vi "2015 INI Loader.vi"() -> (1 "Inches Per Tick":dbl=0.103 format="%.4f", 2 "Gyro 1 Center Voltage":dbl format="%.4f", 3 "Gyro 1 Gain":dbl format="%.4f", 5 "Turn PID gains":T1={"proportional gain (Kc)"=0.015999999999999997, "integral time (Ti, min)"=0.01800000000000001, "derivative time (Td, min)"=0.0} {"proportional gain (Kc)" min=0.0 max=1.0 step=0.001; "integral time (Ti, min)" min=0.0 max=1.0 step=0.001}, 6 "Elevator PID gains":T1={"proportional gain (Kc)"=1.0, "integral time (Ti, min)"=0.01, "derivative time (Td, min)"=0.0} {"derivative time (Td, min)" format="%.3f"; "integral time (Ti, min)" format="%.3f"; "proportional gain (Kc)" format="%.3f"}, 7 "Base PID gains":T1 {"derivative time (Td, min)" format="%.3f"; "integral time (Ti, min)" format="%.3f"; "proportional gain (Kc)" format="%.3f"})   [LabVIEW 2014]
uses:
  PID Typdef.ctl
  <vilib>/Utility/config.llb/Read Key (Double).vi
  <vilib>/Rock Robotics/Network Tables/SD Write String.vi
  <vilib>/Utility/config.llb/NI_LVConfig.lvlib
panel:
  out "ED":dbl
  out "EI":dbl
  out "EP":dbl
  out "TD":dbl
  out "TI":dbl
  out "TP":dbl
  out "BED":dbl
  out "BEI":dbl
  out "BEP":dbl
  out "path":path
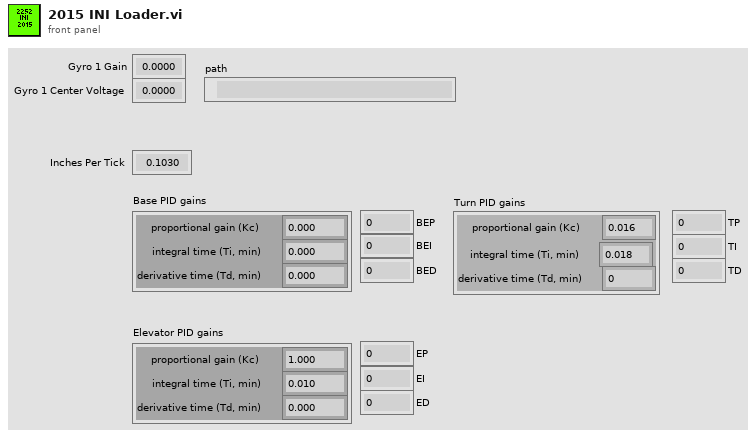
[diagram p1: front panel]
types:
  T1 = cluster{"proportional gain (Kc)":dbl, "integral time (Ti, min)":dbl, "derivative time (Td, min)":dbl}
  T2 = typedef "PID Typdef.ctl" = cluster{"proportional gain (Kc)":dbl, "integral time (Ti, min)":dbl, "derivative time (Td, min)":dbl}
  T3 = typedef "NI_LVConfig.lvlib/Config Data RefNum.ctl" = refnum<k1>
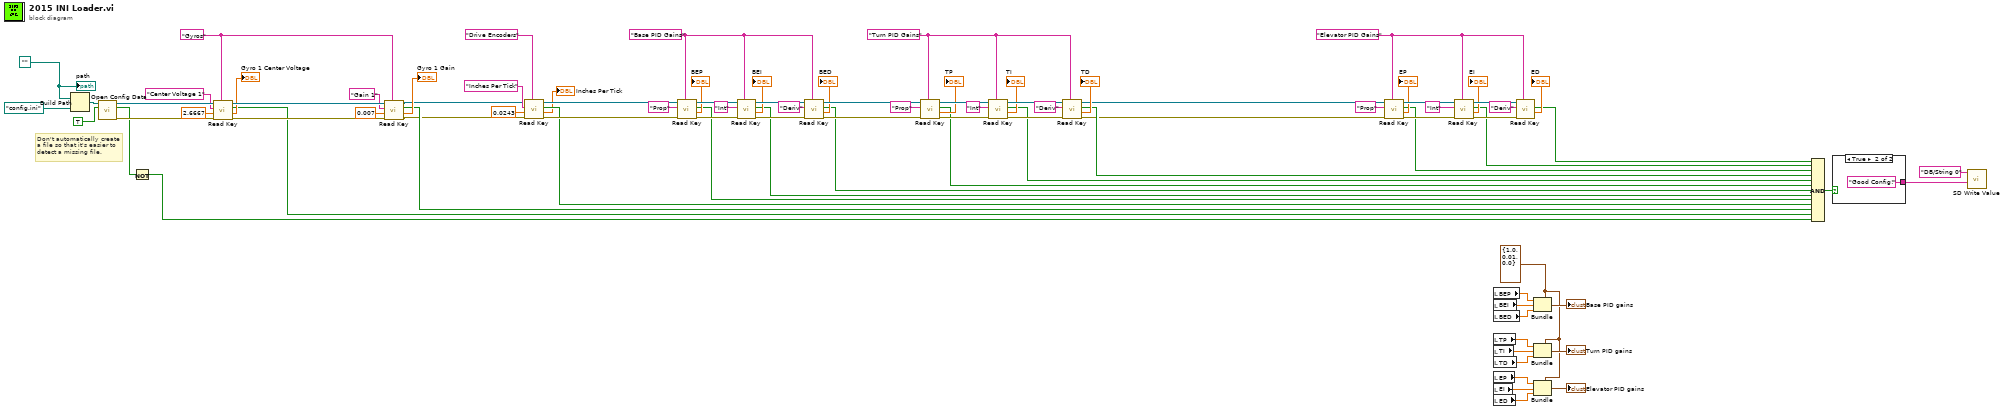
[diagram p0: block diagram]
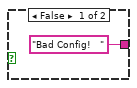
[diagram p2: hidden frame]
diagram:
  w3 = path ""
  w62 = T2 {"proportional gain (Kc)"=1.0, "integral time (Ti, min)"=0.01, "derivative time (Td, min)"=0.0} ("PID Typedef")
  w41 = "Elevator PID Gains" ("section")
  w44 = "Turn PID Gains" ("section")
  w53 = "Base PID Gains" ("section")
  w77 = "Gyros" ("section")
  # "Don't automatically create\na file so that it's easier to\ndetect a missing file."
  n1 = Build Path(base path=w3, name or relative path=path "config.ini" ("configuration file path")) -> (appended path=w89:path)
  n2 = call <vilib>:"Open Config Data.vi"("create file if necessary (T)"=TRUE, "configuration file path"=w89) -> ("error out"=w88:errorcluster, "file created?"=w81:bool, "refnum"=w87:T3)  [unwired: 7 in]
  n3 = Not(x=w81) -> (.not. x?=w69:bool)
  n4 = call-poly <vilib>:"Read Key.vi"("section"=w77, "error in (no error)"=w88, "default value"=2.6667, "key"="Center Voltage 1", "refnum"=w87) -> ("error out"=w84:errorcluster, "value"=→"Gyro 1 Center Voltage":dbl, "found?"=w70:bool, "refnum out"=w83:T3)  [unwired: 3 in]
  n5 = call-poly <vilib>:"Read Key.vi"("section"=w77, "error in (no error)"=w84, "default value"=0.007, "key"="Gain 1", "refnum"=w83) -> ("error out"=w66:errorcluster, "value"=→"Gyro 1 Gain":dbl, "found?"=w71:bool, "refnum out"=w65:T3)  [unwired: 3 in]
  n6 = call-poly <vilib>:"Read Key.vi"("section"="Drive Encoders", "error in (no error)"=w66, "default value"=0.0243, "key"="Inches Per Tick", "refnum"=w65) -> ("error out"=w60:errorcluster, "value"=→"Inches Per Tick":dbl, "found?"=w14:bool, "refnum out"=w59:T3)  [unwired: 3 in]
  n7 = call-poly <vilib>:"Read Key.vi"("section"=w53, "error in (no error)"=w60, "key"="Prop", "refnum"=w59) -> ("error out"=w49:errorcluster, "value"=→"BEP":dbl, "found?"=w13:bool, "refnum out"=w58:T3)  [unwired: 4 in]
  n8 = call-poly <vilib>:"Read Key.vi"("section"=w53, "error in (no error)"=w49, "key"="Int", "refnum"=w58) -> ("error out"=w48:errorcluster, "value"=→"BEI":dbl, "found?"=w12:bool, "refnum out"=w57:T3)  [unwired: 4 in]
  n9 = call-poly <vilib>:"Read Key.vi"("section"=w53, "error in (no error)"=w48, "key"="Deriv", "refnum"=w57) -> ("error out"=w47:errorcluster, "value"=→"BED":dbl, "found?"=w11:bool, "refnum out"=w56:T3)  [unwired: 4 in]
  n10 = call-poly <vilib>:"Read Key.vi"("section"=w44, "error in (no error)"=w47, "key"="Prop", "refnum"=w56) -> ("error out"=w46:errorcluster, "value"=→"TP":dbl, "found?"=w10:bool, "refnum out"=w55:T3)  [unwired: 4 in]
  n11 = call-poly <vilib>:"Read Key.vi"("section"=w44, "error in (no error)"=w46, "key"="Int", "refnum"=w55) -> ("error out"=w45:errorcluster, "value"=→"TI":dbl, "found?"=w9:bool, "refnum out"=w54:T3)  [unwired: 4 in]
  n12 = call-poly <vilib>:"Read Key.vi"("section"=w44, "error in (no error)"=w45, "key"="Deriv", "refnum"=w54) -> ("error out"=w1:errorcluster, "value"=→"TD":dbl, "found?"=w8:bool, "refnum out"=w2:T3)  [unwired: 4 in]
  n13 = call-poly <vilib>:"Read Key.vi"("section"=w41, "error in (no error)"=w1, "key"="Prop", "refnum"=w2) -> ("error out"=w42:errorcluster, "value"=→"EP":dbl, "found?"=w7:bool, "refnum out"=w43:T3)  [unwired: 4 in]
  n14 = call-poly <vilib>:"Read Key.vi"("section"=w41, "error in (no error)"=w42, "key"="Int", "refnum"=w43) -> ("error out"=w39:errorcluster, "value"=→"EI":dbl, "found?"=w6:bool, "refnum out"=w40:T3)  [unwired: 4 in]
  n15 = local read "BEP"() -> (w33:dbl)
  n16 = local read "BEI"() -> (w34:dbl)
  n17 = local read "BED"() -> (w35:dbl)
  n18 = local read "TP"() -> (w20:dbl)
  n19 = local read "TI"() -> (w19:dbl)
  n20 = local read "TD"() -> (w18:dbl)
  n21 = local read "EP"() -> (w16:dbl)
  n22 = local read "EI"() -> (w17:dbl)
  n23 = local read "ED"() -> (w15:dbl)
  n24 = call-poly <vilib>:"Read Key.vi"("section"=w41, "error in (no error)"=w39, "key"="Deriv", "refnum"=w40) -> ("value"=→"ED":dbl, "found?"=w5:bool)  [unwired: 4 in, 2 out]
  n25 = Bundle(cluster=w62, "proportional gain (Kc)"=w33, "integral time (Ti, min)"=w34, "derivative time (Td, min)"=w35) -> (→"Base PID gains":T2)
  n26 = Bundle(cluster=w62, "proportional gain (Kc)"=w20, "integral time (Ti, min)"=w19, "derivative time (Td, min)"=w18) -> (→"Turn PID gains":T2)
  n27 = Bundle(cluster=w62, "proportional gain (Kc)"=w16, "integral time (Ti, min)"=w17, "derivative time (Td, min)"=w15) -> (→"Elevator PID gains":T2)
  n28 = Compound Arithmetic op=AND(w5, w6, w7, w8, w9, w10, w11, w12, w13, w14, w71, w70, w69) -> (w78:bool)
  n29 = case shown="True" w78 {
    tunnel: ["Bad Config!   " ("line text") "Good Config!" ("line text")] -> w68
    frame False {
    }
    frame True {
    }
  }
  n30 = call-poly <vilib>:"SD Write Value.vi"("String"=w68, "Name"="DB/String 0") -> ()  [unwired: 8 in, 2 out]
  "path" <- w3
